vi "Self Test.vi"(8 "error in (no error)":errorcluster, 11 "2525 in":refnum<class "2525.lvclass">) -> (0 "error out":errorcluster, 3 "2525 out":refnum<class "2525.lvclass">)   [LabVIEW 2019, in "2525.lvlib" / "2525.lvclass"]
uses:
  Library/2525.lvclass
  Library/2525.lvclass/2525.ctl
  Accessors/Read Local Resource.vi
  Accessors/Write Local Resource.vi
  builds/Instruments/SwitchMatrix.lvlibp/Library/SwitchMatrix.lvclass
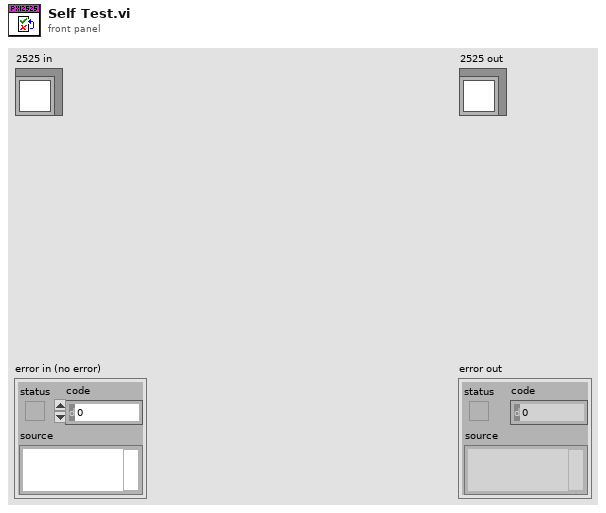
[diagram p1: front panel]
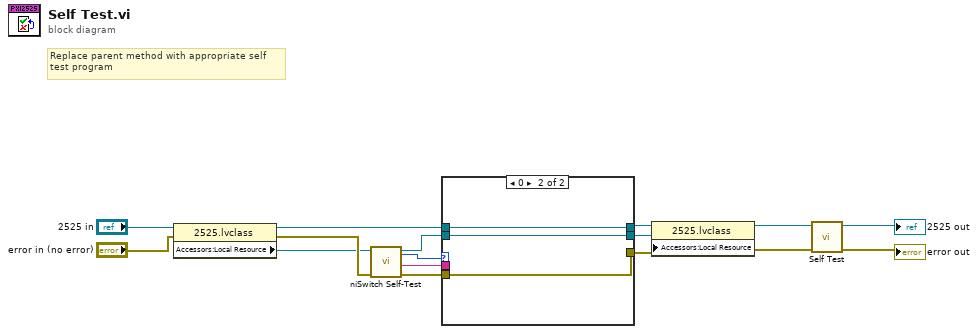
[diagram p0: block diagram]
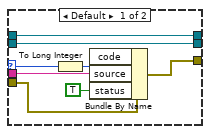
[diagram p2: hidden frame]
diagram:
  # "Replace parent method with appropriate self\ntest program"
  n1 = property class="2525.lvclass"(reference="2525 in", error in="error in (no error)") -> (reference out=w11:refnum<class "2525.lvclass">, error out=w13:errorcluster, "Accessors:Local Resource"=w12:refnum<k15>)
  n2 = call <instrlib>:"niSwitch Self-Test.vi"("error in (no error)"=w13, "instrument handle"=w12) -> ("error out"=w9:errorcluster, "instrument handle out"=w10:refnum<k15>, "self-test message"=w8:string, "self-test result"=w7:i16)  [unwired: 6 in]
  n3 = case shown="0" w7 {
    selector: w7 -> [w18 _]
    tunnel: w10 -> [w19 w25]
    tunnel: w9 -> [w23 w26]
    tunnel: w8 -> [w22 _]
    tunnel: [w20 w26] -> w3
    tunnel: [w19 w25] -> w5
    tunnel: w11 -> [w16 w24]
    tunnel: [w16 w24] -> w6
    frame Default {
      n4 = To Long Integer(number=w18) -> (32bit integer=w17:i32)
      n5 = Bundle By Name(cluster=w23, "code"=w17, "source"=w22, "status"=TRUE) -> (w20:errorcluster)
    }
    frame 0 {
    }
  }
  n6 = property class="2525.lvclass"(reference=w6, "Accessors:Local Resource"=w5) -> (reference out=w4:refnum<class "2525.lvclass">)  [unwired: 1 in, 1 out]
  n7 = call-parent "Self Test.vi"("error in"=w3, "Instruments in"=w4) -> ("error out"=→"error out":errorcluster, "Instruments out"=→"2525 out":refnum<class "2525.lvclass">)  [unwired: 8 in]
